vi "Unconfigure Banana.vi"(8 "error in":errorcluster, 11 "Variety Configured":string) -> (0 "error out":errorcluster)   [LabVIEW 2021, in "Bananas.lvlib"]
uses:
  Bananas.lvlib
  Banana/Banana.lvclass
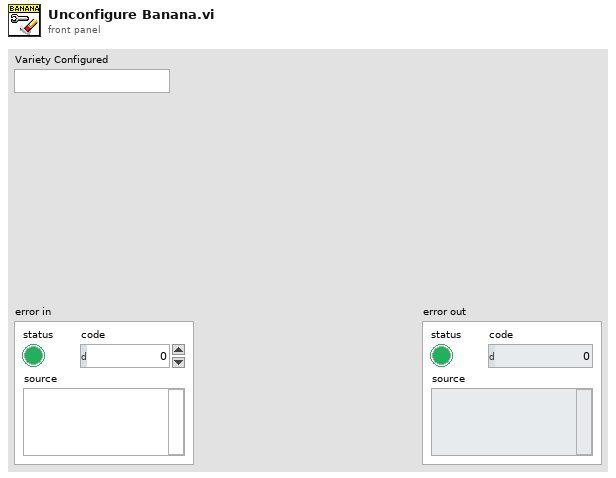
[diagram p1: front panel]
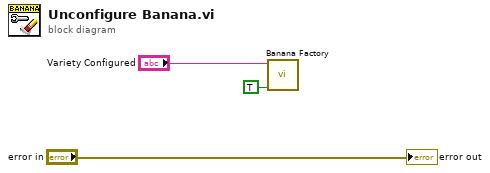
[diagram p0: block diagram]
diagram:
  n1 = call "Banana Factory.vi"("Clear"=TRUE, "Variety"="Variety Configured") -> ()  [unwired: 8 in, 2 out]
  "error out" <- "error in"
